vi "Sub_Initialize_LEMP_with_pred.vi"(3 "Effected DOF":i32, 4 "Stiff":T2, 5 "Mass":T2) -> (0 "Natural freq Cantilever pin":dbl[](array[numeric]), 1 "Natural freq Cantilever":dbl[](array[numeric]), 2 "LEMP":T1)   [LabVIEW 2019]
uses:
  <vilib>/Analysis/Matrix/Datatypes/RealMatrix.ctl
  <vilib>/Analysis/7linalg.llb/Real Generalized Eigenvalues and Vectors.vi
  <vilib>/Analysis/Matrix/Numeric/Conversions/Matrix To Array - RM.vi
  <vilib>/Analysis/Matrix/Numeric/Conversions/Array To Matrix - RA2.vi
  <vilib>/Analysis/NI_AALPro.lvlib
  <vilib>/Analysis/Matrix/NI_Matrix.lvlib
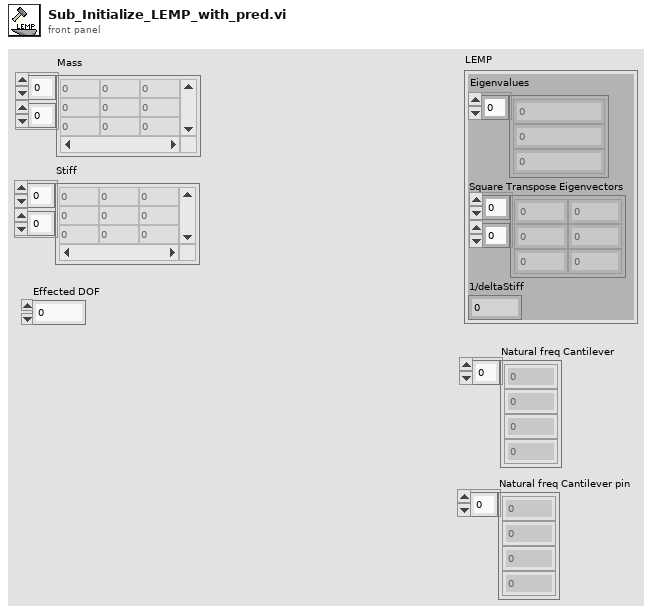
[diagram p1: front panel]
types:
  T1 = cluster{"Eigenvalues":dbl[], "Square Transpose Eigenvectors":dbl[][], "1/deltaStiff":dbl}
  T2 = typedef "NI_Matrix.lvlib/RealMatrix.ctl" = dbl[][]
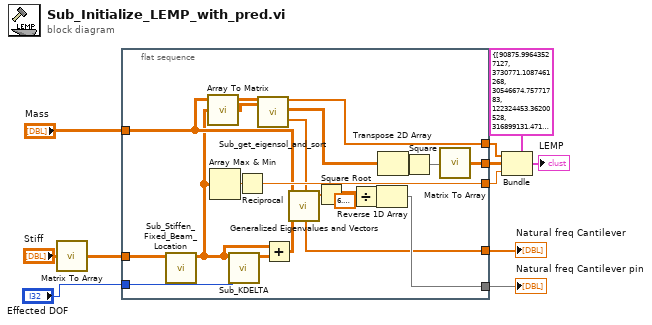
[diagram p0: block diagram]
diagram:
  n1 = call-poly <vilib>:"Matrix To Array.vi"("Real Matrix"="Stiff") -> ("Real 2D Array"=w8:dbl[][])
  n2 = flat-sequence {
    tunnel: [w26] -> w11
    tunnel: [w25] -> w3
    tunnel: [w13] -> w2
    tunnel: [w19] -> w1
    tunnel: "Mass" -> [w18]
    tunnel: "Effected DOF" -> [w17]
    tunnel: w8 -> [w15]
    tunnel: [w14] -> w6
    frame #0 {
      n3 = call "Sub_Stiffen_Fixed_Beam_Location.vi"("Pre-BC Matrix"=w15) -> ("Post-BC Matrix"=w12:dbl[][])  [unwired: 10 in]
      n4 = call-poly <vilib>:"Array To Matrix.vi"("Real 2D Array"=w12) -> ("Real Matrix"=w16:T2)
      n5 = Array Max & Min(array=w12) -> (max value=w21:dbl)  [unwired: 3 out]
      n6 = call "Sub_KDELTA.vi"("Pin-Location"=w17, "Pre-Pin Matrix"=w12) -> ("K12"=w23:dbl[][])  [unwired: 8 in]
      n7 = Reciprocal(x=w21) -> (1/x=w19:dbl)
      n8 = call "Sub_get_eigensol_and_sort.vi"("Mass"=w18, "Stiffness"=w16) -> ("Unsorted Eigenvalues"=w25:dbl[], "Unsorted Eigenvector Matrix"=w24:T2, "Natural frequency"=w14:dbl[])  [unwired: 13 in, 2 out]
      n9 = Add(x=w12, y=w23) -> (x+y=w20:dbl[][])
      n10 = call-poly <vilib>:"Generalized Eigenvalues and Vectors.vi"("B"=w18, "A"=w20) -> ("Eigenvalues"=w30:cdb[])  [unwired: 4 in, 2 out]
      n11 = Square Root(x=w30) -> (sqrt(x)=w29:cdb[])
      n12 = Divide(x=w29, y=6.283185307179586) -> (x/y=w27:cdb[])
      n13 = Reverse 1D Array(array=w27) -> (reversed array=w26:cdb[])
      n14 = Transpose 2D Array(2D array=w24) -> (transposed array=w31:T2)
      n15 = Square(x=w31) -> (x^2=w22:T2)
      n16 = call-poly <vilib>:"Matrix To Array.vi"("Real Matrix"=w22) -> ("Real 2D Array"=w13:dbl[][])
    }
  }
  n17 = Bundle(cluster=T1 {"Eigenvalues"=[90875.99643527127, 3730771.1087461268, 30546674.75771783, 122324453.36200528, 316899131.47196954, 389800029.50389755, 995792500.6195576, 1778378352.4567704, 2935210286.098047, 4581053874.543485, 6838189882.736964, 9842579078.498016, 13744292882.429237, 18708098659.573277, 24913198797.158657, 32553944531.79768, 41840422615.38715, 52998970022.19148, 66272898146.151405, 81923349416.47206, 100230217134.0868, 121493239373.70726, 146033178623.99777, 174193047917.5844, 206339492111.7017, 242864110260.8828, 284184583713.8293, 330745750176.43036, 383019540222.79926, 441504114453.6817, 506719891954.99274, 579200971152.0848, 659474243200.3528, 748016085151.9138, 845147985539.1793, 950772242570.3394, 1063603211663.3796, 1178562417924.1416, 1277742005467.3933, 1657100457470.6738, 1793525840889.8276, 1973135066757.3123, 2181201801841.3132, 2414150445859.6206, 2671853278417.392, 2955448191268.974, 3266686974458.4536, 3607713226917.2134, 3980980609815.778, 4389223418841.7554, 4835448132857.691, 5322932756984.317, 5855227084251.794, 6436149100158.893, 7069773123791.937, 7760404756492.608, 8512536615660.194, 9330777279240.41, 10219743907095.484, 11183906715308.416, 12227371013213.818, 13353580181129.566, 14564921334934.777, 15862215428566.658, 17244076658352.232, 18706134151085.867, 20240124980955.25, 21832893766216.004, 23465373434158.88, 25111673866694.44, 26738466597464.11, 28304914382402.473, 29763436640385.207, 31061599947115.277, 32145343365358.03, 32963547203421.62, 33473582378987.473, 47871301251493.97, 1.476650659083303e+17, 4.071133824147183e+23], "Square Transpose Eigenvectors"=[], "1/deltaStiff"=1e-15} ("LEMP"), "Eigenvalues"=w3, "Square Transpose Eigenvectors"=w2, "1/deltaStiff"=w1) -> (→"LEMP":T1)
  "Natural freq Cantilever pin" <- w11
  "Natural freq Cantilever" <- w6
